vi "Plan Joint Move.vi"(4 "Side":T2=enum."right", 7 "[6Tg]^-1":T1, 8 "queue":refnum<queue>, 9 "Joints":dbl[](array[numeric]), 11 "Goal":T3) -> (0 "0 Speed?":bool, 3 "Label":string)   [LabVIEW 2013]
uses:
  Goal.ctl
  <vilib>/Analysis/Matrix/Datatypes/RealMatrix.ctl
  ROS/Code/SubVIs/BaxterSide.ctl
  <vilib>/Analysis/Matrix/Numeric/Multiply/Multiply - RM,RM.vi
  <vilib>/Analysis/Matrix/NI_Matrix.lvlib
panel:
  out "error out":errorcluster
  in  "stop":bool
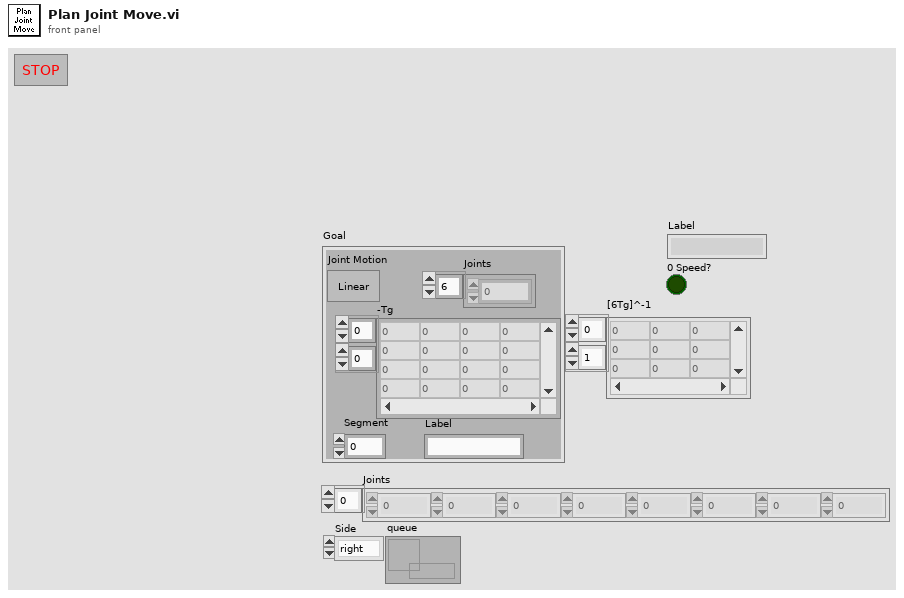
[diagram p1: front panel]
types:
  T1 = typedef "NI_Matrix.lvlib/RealMatrix.ctl" = dbl[][]
  T2 = typedef "BaxterSide.ctl" = enum16{"left", "right"}
  T3 = typedef "Goal.ctl" = cluster{"Segment":dbl, "-Tg":T1, "Joints":dbl[], "Label":string, "Joint Motion":bool}
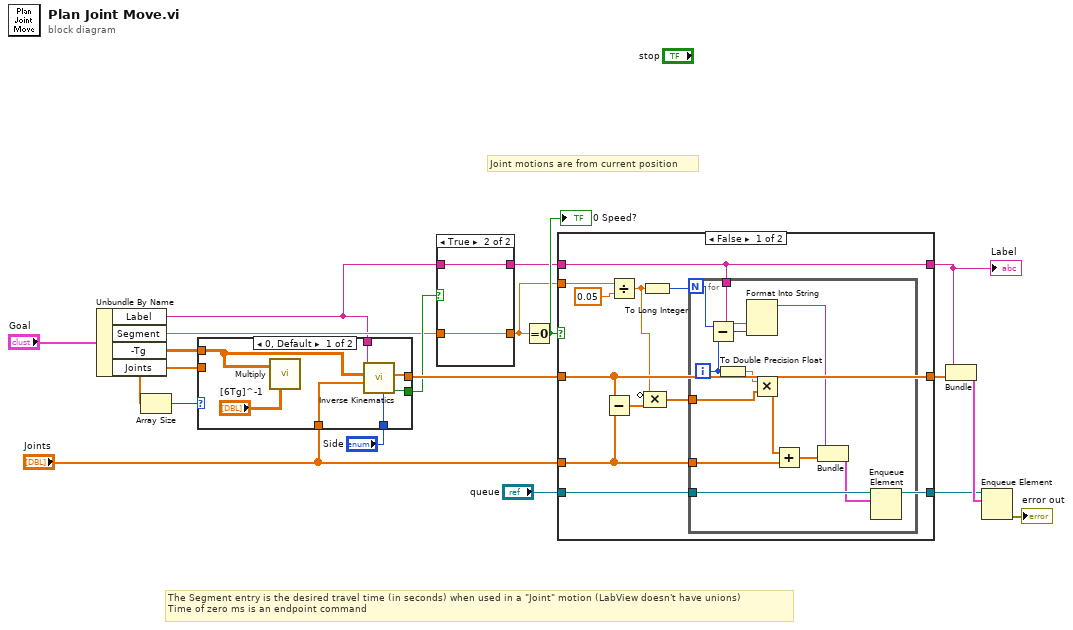
[diagram p0: block diagram]
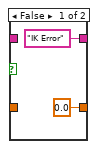
[diagram p2: hidden frame]
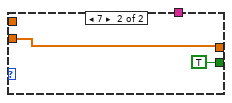
[diagram p4: hidden frame]
diagram:
  # "Joint motions are from current position"
  # "The Segment entry is the desired travel time (in seconds) when used in a \"Joint\" motion (LabView doesn't have unions)\nTime of zero ms is an endpoint command"
  n1 = Unbundle By Name("Goal") -> ("Label"=w2:string, "Segment"=w11:dbl, "-Tg"=w3:T1, "Joints"=w4:dbl[])
  n2 = Array Size(array=w4) -> (size(s)=w5:i32)
  n3 = case shown="0, Default" w5 {
    tunnel: [w26 w27] -> w16
    tunnel: "Joints" -> [w25 _]
    tunnel: [w24 TRUE ("Found")] -> w12
    tunnel: "Side" -> [w23 _]
    tunnel: w4 -> [_ w27]
    tunnel: w3 -> [w21 _]
    tunnel: w2 -> [w20 _]
    frame 0, Default {
      n4 = call-poly <vilib>:"Multiply.vi"("Real Matrix B"="[6Tg]^-1", "Real Matrix A"=w21) -> ()  [unwired: 1 out]
      n5 = call "Inverse Kinematics.vi"("Side"=w23, "Start"=w25, "Goal-matrix"=w21, "Label"=w20) -> ("Found"=w24:bool, "J"=w26:dbl[])  [unwired: 4 in, 2 out]
    }
    frame 7 {
    }
  }
  n6 = case shown="True" w12 {
    tunnel: w2 -> [_ w32]
    tunnel: w11 -> [_ w31]
    tunnel: ["IK Error" ("Label") w32] -> w10
    tunnel: [0.0 ("Speed") w31] -> w9
    frame False {
    }
    frame True {
    }
  }
  n7 = Equal To 0?(x=w9) -> (x = 0?=w17:bool)
  "0 Speed?" <- w17
  n8 = case shown="False" w17 {
    tunnel: w16 -> [w35 w57]
    tunnel: [w35 w57] -> w15
    tunnel: w10 -> [w36 w56]
    tunnel: [w36 w56] -> w14
    tunnel: "queue" -> [w34 w55]
    tunnel: [w34 w55] -> w13
    tunnel: w9 -> [w41 _]
    tunnel: "Joints" -> [w37 _]
    frame False {
      n9 = Subtract(x=w35, y=w37) -> (x-y=w42:dbl[])
      n10 = Divide(x=w41, y=0.05) -> (x/y=w33:dbl)
      n11 = To Long Integer(number=w33) -> (32bit integer=w39:i32)
      n12 = Compound Arithmetic op=MULTIPLY(invert w33, w42) -> (w38:dbl[])
      n13 = for {
        N: w39 -> [w48]
        tunnel: w38 -> [w53]
        tunnel: w37 -> [w51]
        tunnel: w36 -> [w50]
        tunnel: w34 -> [w44]
        i -> [w47]
        n14 = Subtract(x=w48, y=w47) -> (x-y=w49:i32)
        n15 = To Double Precision Float(number=w47) -> (double precision float=w54:dbl)
        n16 = Format Into String(w50, w49) -> (resulting string=w45:string)  [unwired: 3 in, 1 out]
        n17 = Multiply(x=w54, y=w53) -> (x*y=w52:dbl[])
        n18 = Add(x=w52, y=w51) -> (x+y=w46:dbl[])
        n19 = Bundle(w45, w46) -> (w43:cluster{string, dbl[]})  [unwired: 1 in]
        n20 = Enqueue Element(queue=w44, element=w43) -> ()  [unwired: 2 in, 3 out]
      }
    }
    frame True {
    }
  }
  "Label" <- w14
  n21 = Bundle("Label"=w14, "Joints"=w15) -> (w18:cluster{"Label":string, "Joints":dbl[]})  [unwired: 1 in]
  n22 = Enqueue Element(queue=w13, element=w18) -> (error out=→"error out":errorcluster)  [unwired: 2 in, 2 out]
